vi "ReadRecords.vi"(8 "error in (no error)":errorcluster, 10 "Num records to read":i32, 11 "FpgaRef5761 In":refnum<class "FpgaRef5761.lvclass">) -> (0 "error out":errorcluster, 2 "Data":dbl[][](array[numeric]), 3 "FpgaRef5761 Out":refnum<class "FpgaRef5761.lvclass">)   [LabVIEW 2018, in "FpgaRef5761.lvclass"]
uses:
  FpgaRef5761.lvclass
  FpgaRef5761.lvclass/FpgaRef5761.ctl
  <vilib>/Utility/error.llb/Error Cluster From Error Code.vi
  <vilib>/rvi/errors/niLvFpgaAdjustHostInterfaceError.vi
  <vilib>/rvi/interface/nirviMethod/nirviMethod.xnode
  5761 FPGA ref.ctl
  <vilib>/FPGAPlugInAG/Dynamic/niLvFpga_ReadFifo_Dynamic.vi
  <vilib>/rvi/errors/niLvFpgaMergeErrorWithErrorCode.vi
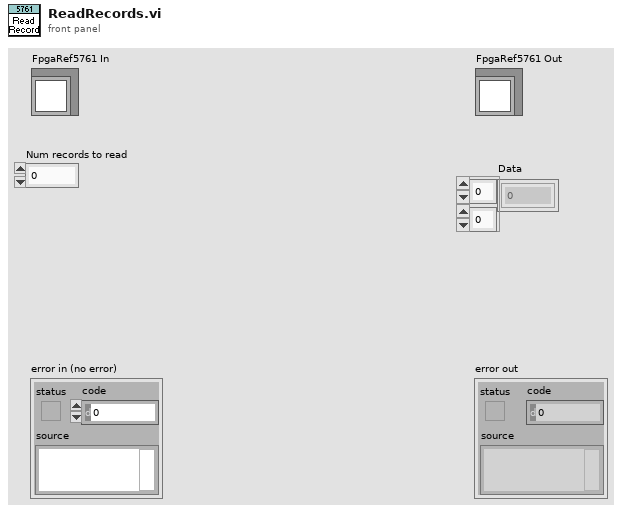
[diagram p1: front panel]
types:
  T1 = typedef "5761 FPGA ref.ctl" = refnum<k20>
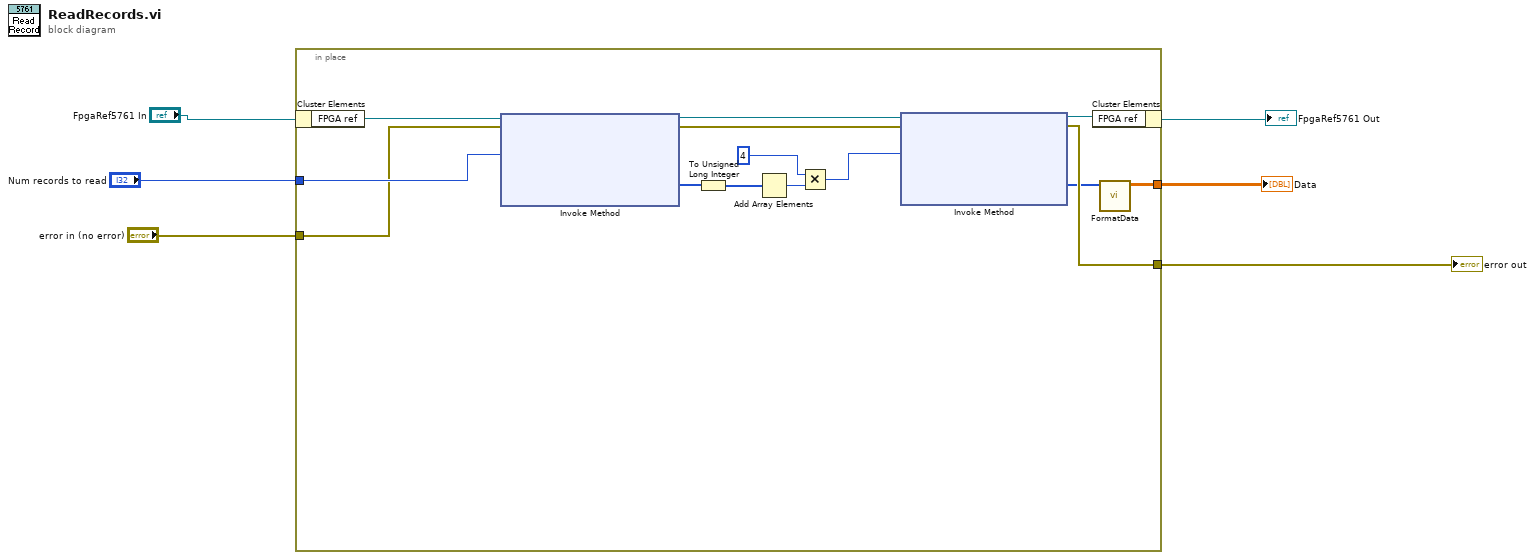
[diagram p0: block diagram]
diagram:
  n1 = in-place {
    in-place-border: "Num records to read" -> [w19]
    in-place-border: "error in (no error)" -> [w18]
    in-place-border: [w10] -> w2
    in-place-border: [w8] -> w1
    n2 = in-place-cluster #1("FpgaRef5761 In") -> ("FPGA ref"=w20:T1)
    n3 = xnode "Invoke Method"("FPGA VI Reference In"=w20, "error in"=w18, "Number of Elements"=w19) -> ("FPGA VI Reference Out"=w13:T1, "error out"=w9:errorcluster, "Data"=w17:u16[])  [unwired: 1 in, 1 out]
    n4 = To Unsigned Long Integer(number=w17) -> (unsigned 32bit integer=w16:u32[])
    n5 = Add Array Elements(numeric array=w16) -> (sum=w15:u32)
    n6 = Multiply(x=u32 4, y=w15) -> (x*y=w12:u32)
    n7 = xnode "Invoke Method"("FPGA VI Reference In"=w13, "error in"=w9, "Number of Elements"=w12) -> ("FPGA VI Reference Out"=w11:T1, "error out"=w8:errorcluster, "Data"=w7:u64[])  [unwired: 1 in, 1 out]
    n8 = in-place-cluster #1("FPGA ref"=w11) -> (→"FpgaRef5761 Out":refnum<class "FpgaRef5761.lvclass">)
    n9 = call "FormatData.vi"("Raw data"=w7) -> ("Scaled"=w10:dbl[][])  [unwired: 10 in]
  }
  "error out" <- w1
  "Data" <- w2
